vi "Binary Serialise Unit Tests.vi"(8 "error in (no error)":errorcluster) -> (0 "error out":errorcluster)   [LabVIEW 2021]
uses:
  Source/Variables/Support/Bool/Var_Bool.lvclass
  C:/New folder/LV_Abstract/LV_Abstract/Source/Abs_Types/Boolean/Abs_Boolean.lvclass
  Source/Variables/Support/Time/Var_Time.lvclass
  C:/New folder/LV_Abstract/LV_Abstract/Source/Abs_Types/Time/Abs_Time.lvclass
  Source/Variables/Support/DBL/Var_DBL.lvclass
  C:/New folder/LV_Abstract/LV_Abstract/Source/Abs_Types/Double Float/Abs_Double Float.lvclass
  Source/Variables/Support/EXT/Var_EXT.lvclass
  C:/New folder/LV_Abstract/LV_Abstract/Source/Abs_Types/Extended Float/Abs_Extended Float.lvclass
  Source/Variables/Support/SGL/Var_SGL.lvclass
  C:/New folder/LV_Abstract/LV_Abstract/Source/Abs_Types/Single Float/Abs_Single Float.lvclass
  Source/Variables/Support/CPLX_DBL/Var_CPLX_DBL.lvclass
  C:/New folder/LV_Abstract/LV_Abstract/Source/Abs_Types/Complex Double Float/Abs_Complex Double Float.lvclass
  Source/Variables/Support/CPLX_EXT/Var_CPLX_EXT.lvclass
  C:/New folder/LV_Abstract/LV_Abstract/Source/Abs_Types/Complex Extended Float/Abs_Complex Extended Float.lvclass
  Source/Variables/Support/CPLX_SGL/Var_CPLX_SGL.lvclass
  C:/New folder/LV_Abstract/LV_Abstract/Source/Abs_Types/Complex Single Float/Abs_Complex Single Float.lvclass
  Source/Variables/Support/I8/Var_I8.lvclass
  C:/New folder/LV_Abstract/LV_Abstract/Source/Abs_Types/I8 Integer/Abs_I8 Integer.lvclass
  Source/Variables/Support/I16/Var_I16.lvclass
  C:/New folder/LV_Abstract/LV_Abstract/Source/Abs_Types/I16 Integer/Abs_I16 Integer.lvclass
  Source/Variables/Support/I32/Var_I32.lvclass
  C:/New folder/LV_Abstract/LV_Abstract/Source/Abs_Types/I32 Integer/Abs_I32 Integer.lvclass
  Source/Variables/Support/I64/Var_I64.lvclass
  C:/New folder/LV_Abstract/LV_Abstract/Source/Abs_Types/I64 Integer/Abs_I64 Integer.lvclass
  Source/Variables/Support/U8/Var_U8.lvclass
  C:/New folder/LV_Abstract/LV_Abstract/Source/Abs_Types/U8 Integer/Abs_U8 Integer.lvclass
  Source/Variables/Support/U16/Var_U16.lvclass
  C:/New folder/LV_Abstract/LV_Abstract/Source/Abs_Types/U16 Integer/Abs_U16 Integer.lvclass
  Source/Variables/Support/U32/Var_U32.lvclass
  C:/New folder/LV_Abstract/LV_Abstract/Source/Abs_Types/U32 Integer/Abs_U32 Integer.lvclass
  Source/Variables/Support/U64/Var_U64.lvclass
  C:/New folder/LV_Abstract/LV_Abstract/Source/Abs_Types/U64 Integer/Abs_U64 Integer.lvclass
  Source/Variables/Support/STR/Var_Str.lvclass
  C:/New folder/LV_Abstract/LV_Abstract/Source/Abs_Types/String/Abs_String.lvclass
  ca769228-3f6b-44de-b648-1211edc1de6f.vi
  68a00c68-b0c6-4040-86a2-fcdf1db70f32.vi
  db6b35eb-d347-4d3a-ac23-2f99500d409c.vi
  30870fdf-b604-42f5-a54e-914a7d9e3a9a.vi
  594ac9dd-d076-4f37-a919-b5c684938b95.vi
  8bf99668-d56e-4743-a278-e235c4771389.vi
  c2e982a9-ecd1-433a-8c72-e16931f7f522.vi
  d3cdd1a4-70fd-4048-a5a4-8ece0f5ecdf9.vi
  3b8772d0-f461-46f2-8891-b0a3550c052f.vi
  c08e42a7-1bee-47e8-b921-e81a350e6795.vi
  d403f331-bad6-44df-8bad-8f8f1f3d7878.vi
  4e41df67-4db3-4918-ae50-3e44ec9186ad.vi
  7dd7e505-7472-44c2-9e9d-c36db157814c.vi
  3618cccf-2fc3-45cf-94a0-da3c55d2829a.vi
  7502618b-ff32-4a4e-84fd-a92dfc0de9b7.vi
  e858a5ee-0651-4eaf-b121-e9aada9234b5.vi
  Source/Abs_Types/Abs_Simple_Read.vi
  Source/Abs_Types/Boolean/Simple Read.vi
  Source/Variables/Abs_Init_Variable.vi
  Source/Variables/Support/Bool/Support/Init_Simple_Var.vi
  Source/Abs_Types/String/Simple Read.vi
  Source/Variables/Support/STR/Support/Init_Simple_Var.vi
  Source/Abs_Types/Time/Simple Read.vi
  Source/Variables/Support/Time/Support/Init_Simple_Var.vi
  Source/Abs_Types/Double Float/Simple Read.vi
  Source/Variables/Support/DBL/Support/Init_Simple_Var.vi
  Source/Abs_Types/Extended Float/Simple Read.vi
  Source/Variables/Support/EXT/Support/Init_Simple_Var.vi
  Source/Abs_Types/Single Float/Simple Read.vi
  Source/Variables/Support/SGL/Support/Init_Simple_Var.vi
  Source/Variables/Support/CPLX_DBL/Support/Init_Simple_Var.vi
  Source/Variables/Support/CPLX_EXT/Support/Init_Simple_Var.vi
  Source/Variables/Support/CPLX_SGL/Support/Init_Simple_Var.vi
  Source/Abs_Types/I8 Integer/Simple Read.vi
  Source/Variables/Support/I8/Support/Init_Simple_Var.vi
  Source/Abs_Types/I16 Integer/Simple Read.vi
  Source/Variables/Support/I16/Support/Init_Simple_Var.vi
  Source/Abs_Types/I32 Integer/Simple Read.vi
  Source/Variables/Support/I32/Support/Init_Simple_Var.vi
  Source/Abs_Types/I64 Integer/Simple Read.vi
  Source/Variables/Support/I64/Support/Init_Simple_Var.vi
  Source/Abs_Types/U8 Integer/Simple Read.vi
  Source/Variables/Support/U8/Support/Init_Simple_Var.vi
  Source/Abs_Types/U16 Integer/Simple Read.vi
  Source/Variables/Support/U16/Support/Init_Simple_Var.vi
  Source/Abs_Types/U32 Integer/Simple Read.vi
  Source/Variables/Support/U32/Support/Init_Simple_Var.vi
  Source/Abs_Types/U64 Integer/Simple Read.vi
  Source/Variables/Support/U64/Support/Init_Simple_Var.vi
  <vilib>/Utility/Data Type/Get Type Information.vi
  <vilib>/addons/_JKI Toolkits/Caraya/classes/Test/Define Test.vi
  <vilib>/addons/_JKI Toolkits/Caraya/classes/Assert/Assert.vi
  <vilib>/addons/_JKI Toolkits/Caraya/classes/Assert/Assert Equal Value_Variant.vi
  <vilib>/addons/_JKI Toolkits/Caraya/classes/Assert/Assert Equal Type_Variant.vi
  Source/Abs_Types/Complex Double Float/Simple Read.vi
  Source/Abs_Types/Complex Extended Float/Simple Read.vi
  Source/Abs_Types/Complex Single Float/Simple Read.vi
  Source/Abs_Types/Boolean/Abs_Boolean.lvclass
  Source/Abs_Types/String/Abs_String.lvclass
  Source/Abs_Types/Time/Abs_Time.lvclass
  Source/Abs_Types/Double Float/Abs_Double Float.lvclass
  Source/Abs_Types/Extended Float/Abs_Extended Float.lvclass
  Source/Abs_Types/Single Float/Abs_Single Float.lvclass
  Source/Abs_Types/I8 Integer/Abs_I8 Integer.lvclass
  Source/Abs_Types/I16 Integer/Abs_I16 Integer.lvclass
  Source/Abs_Types/I32 Integer/Abs_I32 Integer.lvclass
  Source/Abs_Types/I64 Integer/Abs_I64 Integer.lvclass
  Source/Abs_Types/U8 Integer/Abs_U8 Integer.lvclass
  Source/Abs_Types/U16 Integer/Abs_U16 Integer.lvclass
  Source/Abs_Types/U32 Integer/Abs_U32 Integer.lvclass
  Source/Abs_Types/U64 Integer/Abs_U64 Integer.lvclass
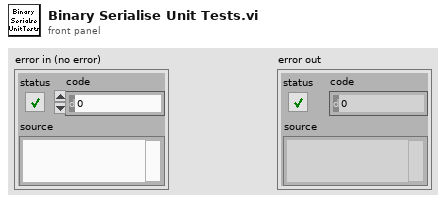
[diagram p1: front panel]
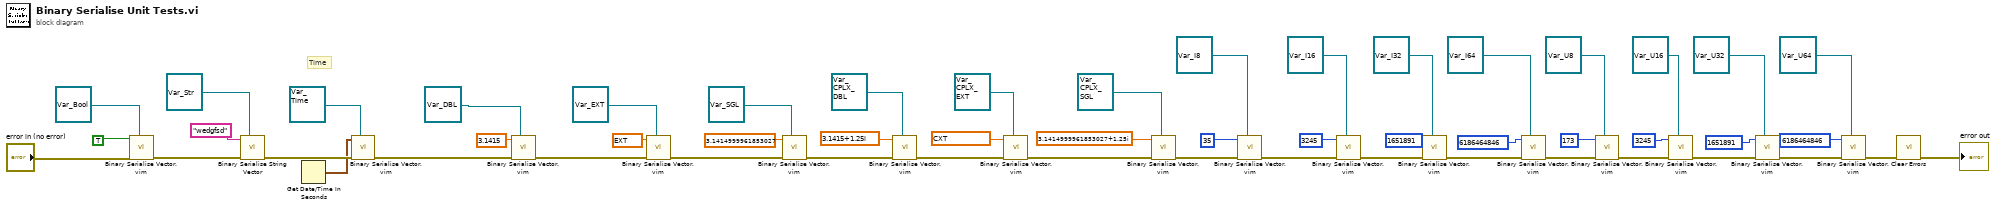
[diagram p0: block diagram]
diagram:
  # "Time"
  n1 = call "Binary Serialise Vector.vim"("Expected Class"=refnum<class "Var_Bool.lvclass"> refnum ("Var_Bool.lvclass"), "error in (no error)"="error in (no error)", "Test Value"=TRUE) -> ("error out"=w46:errorcluster)  [unwired: 8 in]
  n2 = call "Binary Serialise String Vector.vi"("Expected Class"=refnum<class "Var_Str.lvclass"> refnum, "error in (no error)"=w46, "Test Value"="wedgfsd") -> ("error out"=w45:errorcluster)  [unwired: 8 in]
  n3 = Get Date/Time In Seconds() -> (seconds since 1Jan1904=w43:timestamp)
  n4 = call "Binary Serialise Vector.vim"("Expected Class"=refnum<class "Var_Time.lvclass"> refnum ("Var_Time.lvclass"), "error in (no error)"=w45, "Test Value"=w43) -> ("error out"=w44:errorcluster)  [unwired: 8 in]
  n5 = call "Binary Serialise Vector.vim"("Expected Class"=refnum<class "Var_DBL.lvclass"> refnum ("Var_DBL.lvclass"), "error in (no error)"=w44, "Test Value"=3.1415) -> ("error out"=w51:errorcluster)  [unwired: 8 in]
  n6 = call "Binary Serialise Vector.vim"("Expected Class"=refnum<class "Var_EXT.lvclass"> refnum ("Var_EXT.lvclass"), "error in (no error)"=w51, "Test Value"=ext 3.1414999999999999999) -> ("error out"=w48:errorcluster)  [unwired: 8 in]
  n7 = call "Binary Serialise Vector.vim"("Expected Class"=refnum<class "Var_SGL.lvclass"> refnum ("Var_SGL.lvclass"), "error in (no error)"=w48, "Test Value"=sgl 3.1415) -> ("error out"=w42:errorcluster)  [unwired: 8 in]
  n8 = call "Binary Serialise Vector.vim"("Expected Class"=refnum<class "Var_CPLX_DBL.lvclass"> refnum ("Var_CPLX_DBL.lvclass"), "error in (no error)"=w42, "Test Value"=cdb 3.1415+1.25i) -> ("error out"=w39:errorcluster)  [unwired: 8 in]
  n9 = call "Binary Serialise Vector.vim"("Expected Class"=refnum<class "Var_CPLX_EXT.lvclass"> refnum ("Var_CPLX_EXT.lvclass"), "error in (no error)"=w39, "Test Value"=cxt 3.1415+1.25i) -> ("error out"=w37:errorcluster)  [unwired: 8 in]
  n10 = call "Binary Serialise Vector.vim"("Expected Class"=refnum<class "Var_CPLX_SGL.lvclass"> refnum ("Var_CPLX_SGL.lvclass"), "error in (no error)"=w37, "Test Value"=csg 3.1415+1.25i) -> ("error out"=w36:errorcluster)  [unwired: 8 in]
  n11 = call "Binary Serialise Vector.vim"("Expected Class"=refnum<class "Var_I8.lvclass"> refnum ("Var_I8.lvclass"), "error in (no error)"=w36, "Test Value"=i8 35) -> ("error out"=w33:errorcluster)  [unwired: 8 in]
  n12 = call "Binary Serialise Vector.vim"("Expected Class"=refnum<class "Var_I16.lvclass"> refnum ("Var_I16.lvclass"), "error in (no error)"=w33, "Test Value"=i16 3245) -> ("error out"=w31:errorcluster)  [unwired: 8 in]
  n13 = call "Binary Serialise Vector.vim"("Expected Class"=refnum<class "Var_I32.lvclass"> refnum ("Var_I32.lvclass"), "error in (no error)"=w31, "Test Value"=1651891) -> ("error out"=w30:errorcluster)  [unwired: 8 in]
  n14 = call "Binary Serialise Vector.vim"("Expected Class"=refnum<class "Var_I64.lvclass"> refnum ("Var_I64.lvclass"), "error in (no error)"=w30, "Test Value"=i64 6186464846) -> ("error out"=w27:errorcluster)  [unwired: 8 in]
  n15 = call "Binary Serialise Vector.vim"("Expected Class"=refnum<class "Var_U8.lvclass"> refnum ("Var_U8.lvclass"), "error in (no error)"=w27, "Test Value"=u8 173) -> ("error out"=w26:errorcluster)  [unwired: 8 in]
  n16 = call "Binary Serialise Vector.vim"("Expected Class"=refnum<class "Var_U16.lvclass"> refnum ("Var_U16.lvclass"), "error in (no error)"=w26, "Test Value"=u16 3245) -> ("error out"=w24:errorcluster)  [unwired: 8 in]
  n17 = call "Binary Serialise Vector.vim"("Expected Class"=refnum<class "Var_U32.lvclass"> refnum ("Var_U32.lvclass"), "error in (no error)"=w24, "Test Value"=u32 1651891) -> ("error out"=w22:errorcluster)  [unwired: 8 in]
  n18 = call "Binary Serialise Vector.vim"("Expected Class"=refnum<class "Var_U64.lvclass"> refnum ("Var_U64.lvclass"), "error in (no error)"=w22, "Test Value"=u64 6186464846) -> ("error out"=w20:errorcluster)  [unwired: 8 in]
  n19 = call <vilib>:"Clear Errors.vi"("error in (no error)"=w20) -> ("error out"=→"error out":errorcluster)  [unwired: 5 in, 1 out]
